vi "Test Process Request Returns when Process Stopped.vi"(8 "error in (no error)":errorcluster, 11 "Process Test In":refnum<class "Process Test.lvclass">) -> (0 "error out":errorcluster, 3 "Process Test Out":refnum<class "Process Test.lvclass">)   [LabVIEW 2020, in "Process Test.lvclass"]
uses:
  Process Test.lvclass
  Mock Process/Mock Process.lvclass
  <vilib>/Asteme/LUnit/Test Case.lvclass
  Support/Framework Test Support.lvlib
  C:/Users/anton/Documents/GitHub/Triarc-Framework/source/Framework Test/Base Class Test/Base Test.lvclass
  C:/Program Files (x86)/National Instruments/LabVIEW 2020/vi.lib/Asteme/LUnit/Test Case.lvclass
  C:/Users/anton/Documents/GitHub/Triarc-Framework/source/Framework Test/Process Test/Process Test.lvclass
  Framework/Process/Process.lvclass
  C:/Users/anton/Documents/GitHub/Triarc-Framework/source/Framework/Process/Process.lvclass
  C:/Users/anton/Documents/GitHub/Triarc-Framework/source/Framework/Base/Base.lvclass
  C:/Users/anton/Documents/GitHub/Triarc-Framework/source/Framework/Configuration File/Configuration File.lvclass
  C:/Users/anton/Documents/GitHub/Triarc-Framework/source/Framework/Error Handler Interface/Error Handler Interface.lvclass
  C:/Users/anton/Documents/GitHub/Triarc-Framework/source/Framework Test/Mock Process/Mock Process.lvclass
  C:/Users/anton/Documents/GitHub/Triarc-Framework/source/Framework/Helper Loop/Helper Loop.lvclass
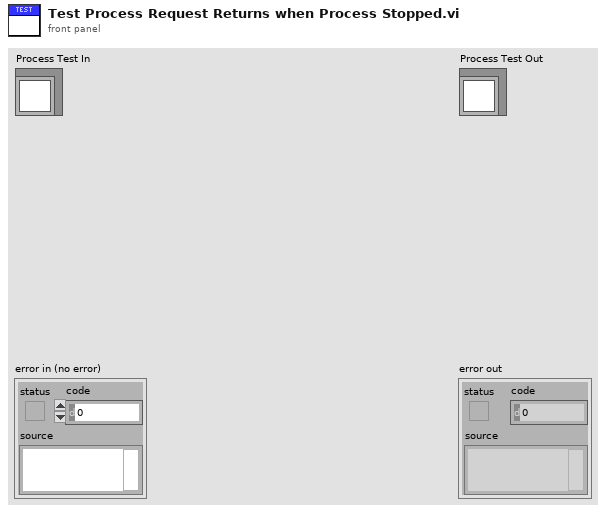
[diagram p1: front panel]
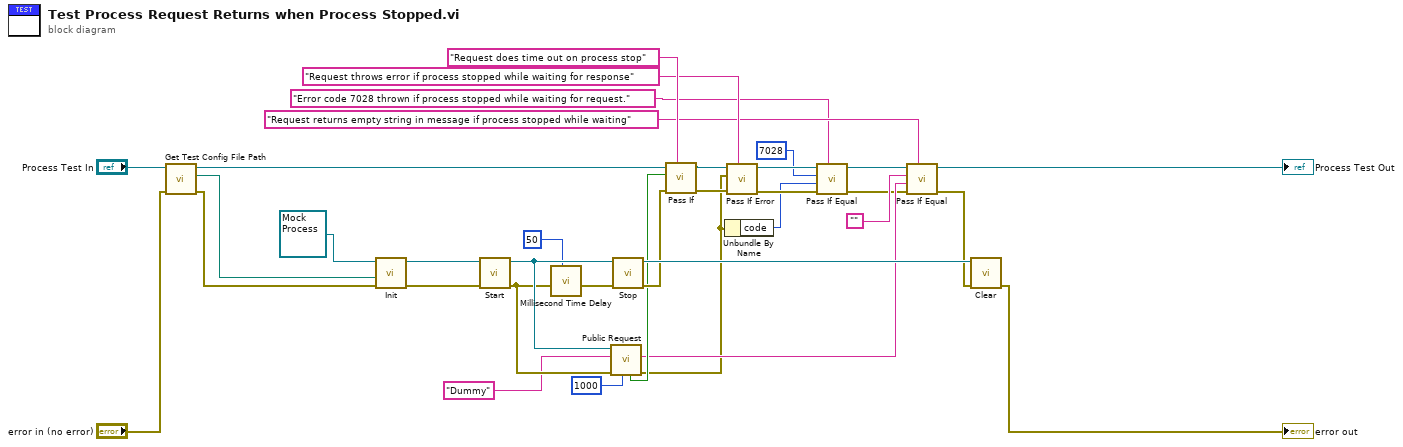
[diagram p0: block diagram]
diagram:
  n1 = call-dynamic "Get Test Config File Path.vi"("error in (no error)"="error in (no error)", "Base Class Test in"="Process Test In") -> ("error out"=w27:errorcluster, "Test config path"=w28:path, "Base Class Test out"=w30:refnum<class "Process Test.lvclass">)  [unwired: 7 in]
  n2 = call-dynamic "Init.vi"("error in (no error)"=w27, "Config File Path"=w28, "Mock Process In"=refnum<class "Mock Process.lvclass"> refnum ("Mock Process.lvclass")) -> ("error out"=w31:errorcluster, "Mock Process Out"=w32:refnum<class "Mock Process.lvclass">)  [unwired: 7 in]
  n3 = call "Start.vi"("error in (no error)"=w31, "Process In"=w32) -> ("error out"=w22:errorcluster, "Process Out"=w23:refnum<class "Mock Process.lvclass">)  [unwired: 8 in]
  n4 = call "Millisecond Time Delay.vi"("milliseconds to wait"=u32 50, "error in (no error)"=w22) -> ("error out"=w2:errorcluster)  [unwired: 7 in]
  n5 = call "Public Request.vi"("timeout in ms"=1000, "error in (no error)"=w22, "Request Message"="Dummy", "Mock Process In"=w23) -> ("error out"=w7:errorcluster, "Response Message"=w15:string, "Timed out?"=w20:bool)  [unwired: 3 in, 2 out]
  n6 = call "Stop.vi"("error in (no error)"=w2, "Process In"=w23) -> ("error out"=w34:errorcluster, "Process Out"=w35:refnum<class "Mock Process.lvclass">)  [unwired: 7 in, 1 out]
  n7 = call <vilib>:"Pass If.vi"("Description"="Request does time out on process stop", "error in (no error)"=w34, "Pass?"=w20, "Test Case In"=w30) -> ("error out"=w19:errorcluster, "Test Case Out"=w26:refnum<class "Process Test.lvclass">)  [unwired: 6 in]
  n8 = Unbundle By Name(w7) -> ("code"=w6:i32)
  n9 = call <vilib>:"Pass If Error.vi"("Description"="Request throws error if process stopped while waiting for response", "error in (no error)"=w19, "Assert error"=w7, "Test Case In"=w26) -> ("error out"=w9:errorcluster, "Test Case Out"=w17:refnum<class "Process Test.lvclass">)  [unwired: 6 in]
  n10 = call <vilib>:"Pass If Equal.vi"("Description"="Error code 7028 thrown if process stopped while waiting for request.", "error in (no error)"=w9, "Actual"=w6, "Expected"=7028 ("code"), "Test Case In"=w17) -> ("error out"=w8:errorcluster, "Test Case Out"=w10:refnum<class "Process Test.lvclass">)  [unwired: 5 in]
  n11 = call <vilib>:"Pass If Equal.vi"("Description"="Request returns empty string in message if process stopped while waiting", "error in (no error)"=w8, "Actual"=w15, "Expected"="", "Test Case In"=w10) -> ("error out"=w18:errorcluster, "Test Case Out"=→"Process Test Out":refnum<class "Process Test.lvclass">)  [unwired: 5 in]
  n12 = call-dynamic "Clear.vi"("error in (no error)"=w18, "Mock Process In"=w35) -> ("error out"=→"error out":errorcluster)  [unwired: 8 in, 1 out]
